vi "Add Update Key.vi"(8 "error in (no error)":errorcluster, 9 "Value":string, 10 "Key":string, 11 "Configuration in":refnum<class "Configuration.lvclass">) -> (0 "error out":errorcluster, 3 "Configuration out":refnum<class "Configuration.lvclass">)   [LabVIEW 2023, in "Configuration.lvlib" / "Configuration.lvclass"]
uses:
  Library/Configuration.lvclass
  Library/Configuration.lvclass/Configuration.ctl
  <vilib>/Utility/config.llb/NI_LVConfig.lvlib
  <vilib>/Utility/config.llb/Write Key (String).vi
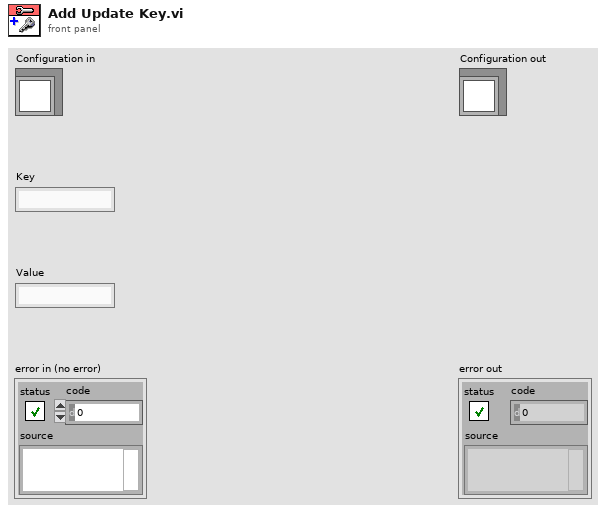
[diagram p1: front panel]
types:
  T1 = typedef "NI_LVConfig.lvlib/Config Data RefNum.ctl" = refnum<k1>
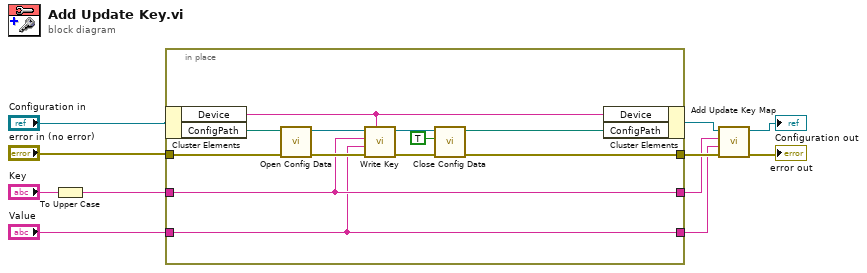
[diagram p0: block diagram]
diagram:
  n1 = To Upper Case(1:"Key") -> (0:w8:string)
  n2 = in-place {
    in-place-border: [w16] -> w4
    in-place-border: "error in (no error)" -> [w15]
    in-place-border: w8 -> [w13]
    in-place-border: "Value" -> [w12]
    in-place-border: [w13] -> w2
    in-place-border: [w12] -> w1
    n3 = in-place-cluster #1("Configuration in") -> ("Device"=w21:string, "ConfigPath"=w20:path)
    n4 = call <vilib>:"Open Config Data.vi"("error in (no error)"=w15, "configuration file path"=w20) -> ("error out"=w18:errorcluster, "refnum"=w23:T1)  [unwired: 7 in, 1 out]
    n5 = call-poly <vilib>:"Write Key.vi"("section"=w21, "error in (no error)"=w18, "value"=w12, "key"=w13, "refnum"=w23) -> ("error out"=w17:errorcluster, "refnum out"=w22:T1)  [unwired: 4 in, 1 out]
    n6 = call <vilib>:"Close Config Data.vi"("error in (no error)"=w17, "write file if changed (T)"=TRUE, "refnum"=w22) -> ("error out"=w16:errorcluster, "file path"=w19:path)  [unwired: 7 in]
    n7 = in-place-cluster #1("Device"=w21, "ConfigPath"=w19) -> (w6:refnum<class "Configuration.lvclass">)
  }
  n8 = call "Add Update Key Map.vi"("error in (no error)"=w4, "Value"=w1, "Key"=w2, "Configuration in"=w6) -> ("error out"=→"error out":errorcluster, "Configuration out"=→"Configuration out":refnum<class "Configuration.lvclass">)  [unwired: 6 in]
